vi "HandleCatch.vi"(7 "InitState":T1=enum."Catch", 8 "error in (no error)":errorcluster, 11 "Toggle?":bool) -> (0 "error out":errorcluster, 3 "State":T1=enum."Catch")   [LabVIEW 2013]
uses:
  CatchAction.ctl
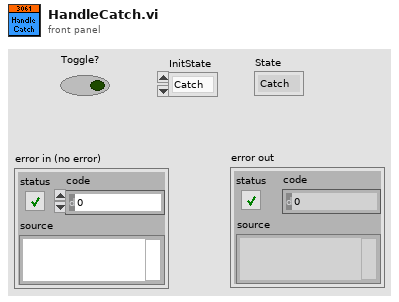
[diagram p1: front panel]
types:
  T1 = typedef "CatchAction.ctl" = enum16{"PreCatch", "Catch", "Stop"}
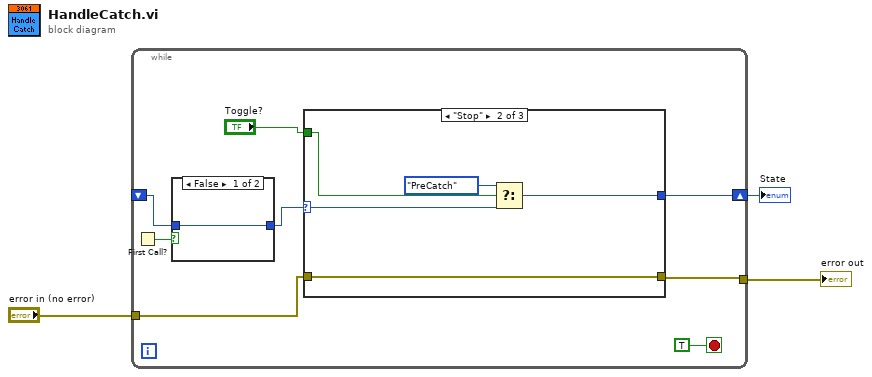
[diagram p0: block diagram]
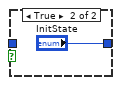
[diagram p2: hidden frame]
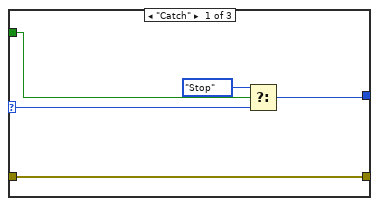
[diagram p3: hidden frame]
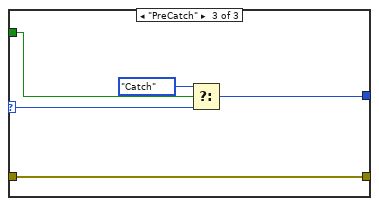
[diagram p4: hidden frame]
diagram:
  n1 = while {
    tunnel: "error in (no error)" -> [w9]
    tunnel: [w8] -> w2
    shift-right: [w6] -> w1
    shift-left: _ -> [w5]
    stop <- TRUE stop-if-true
    n2 = First Call?() -> (First Call?: T/F=w10:bool)
    n3 = case shown="False" w10 {
      tunnel: [w12 "InitState"] -> w7
      tunnel: w5 -> [w12 _]
      frame False {
      }
      frame True {
      }
    }
    n4 = case shown="\"Stop\"" w7 {
      selector: w7 -> [w18 w22 w28]
      tunnel: w9 -> [w17 w23 w24]
      tunnel: [w17 w23 w24] -> w8
      tunnel: "Toggle?" -> [w16 w20 w27]
      tunnel: [w14 w21 w25] -> w6
      frame "Catch" {
        n5 = Select(t=CatchAction."Stop", s=w16, f=w18) -> (s? t:f=w14:T1)
      }
      frame "Stop" {
        n6 = Select(t=CatchAction."PreCatch", s=w20, f=w22) -> (s? t:f=w21:T1)
      }
      frame "PreCatch" {
        n7 = Select(t=CatchAction."Catch", s=w27, f=w28) -> (s? t:f=w25:T1)
      }
    }
  }
  "error out" <- w2
  "State" <- w1
